vi "vms_getSample_M2.vi"(8 "error in (no error)":errorcluster, 11 "M2_Ctl":T1) -> (0 "error out":errorcluster, 2 "function return":i32, 3 "M2_Ctl out":T1)   [LabVIEW 2016, in "SALLV_vms.lvlib"]
doc: "int vms_shm_getSample_M2LV(vms_M2LV *M2_Ctl );"
uses:
  SALLV_vms.lvlib
  DataTypes/M2.ctl
  SALLV_vms.so
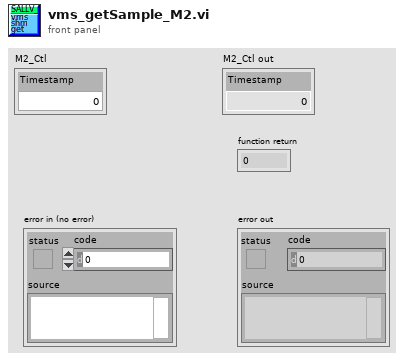
[diagram p1: front panel]
types:
  T1 = typedef "SALLV_vms.lvlib/M2.ctl" = cluster{"Timestamp":dbl}
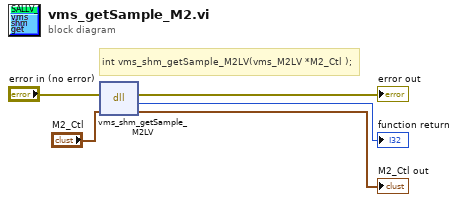
[diagram p0: block diagram]
diagram:
  # "int vms_shm_getSample_M2LV(vms_M2LV *M2_Ctl );"
  n1 = dll-call lib="opt/CODE/SALLV_vms/SALLV_vms.*" fn="vms_shm_getSample_M2LV"(error in="error in (no error)", "M2_Ctl"="M2_Ctl") -> (error out=→"error out":errorcluster, →"function return":i32, "M2_Ctl"=→"M2_Ctl out":T1)  [unwired: 2 in, 1 out]
